vi "Draw Coord Point.vi"(5 "Marker Options":T3={"Color"=3784, "pen"={"Width"=2, "Style"=enum."Solid"}, "font"={"Font Name"="Arial", "Size"=16, "Strikeout?"=FALSE, "Italic?"=FALSE, "Underline?"=FALSE, "Outline?"=FALSE, "Shadow?"=FALSE, "Bold?"=FALSE, "FontColor"=3784}, "caption"=""}, 7 "radius":i16=5, 8 "error in (no error)":errorcluster, 10 "XY":T2, 11 "GarphView in":refnum<class "GarphView.lvclass">) -> (0 "error out":errorcluster, 3 "GarphView out":refnum<class "GarphView.lvclass">)   [LabVIEW 2020, in "GarphView.lvlib" / "GarphView.lvclass"]
uses:
  GarphView.lvclass
  Coords Point.ctl
  <vilib>/Utility/miscctls.llb/LVPoint32TypeDef.ctl
panel:
  out "Coords 2":T1
  out "Coords":T1
  out "XY Graph":cluster{"X":dbl, "Y":dbl}[](graph)
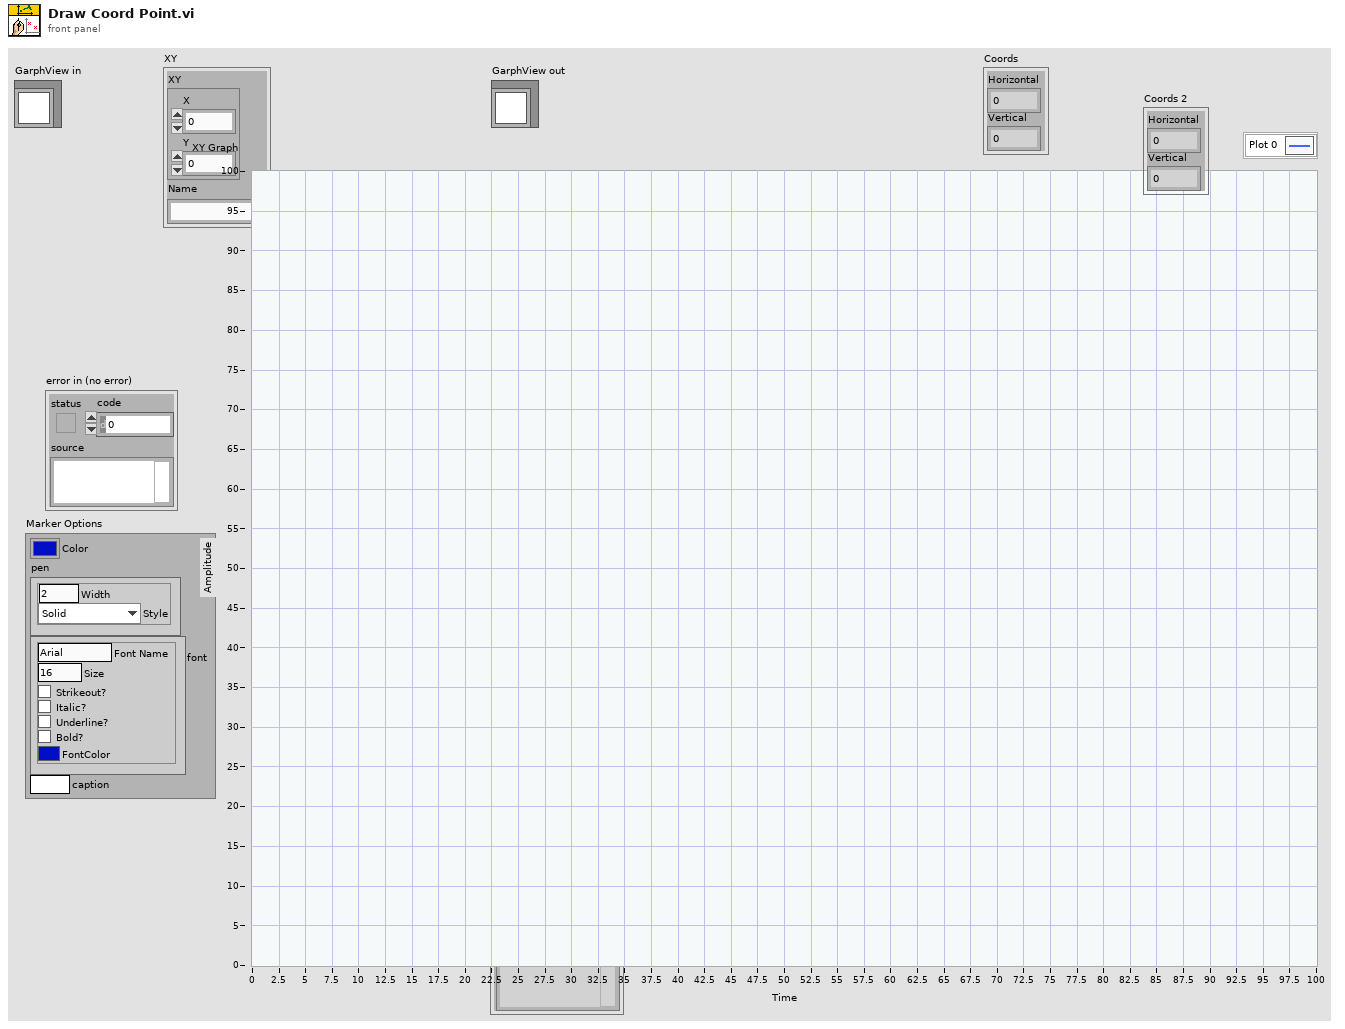
[diagram p1: front panel]
types:
  T1 = typedef "LVPoint32TypeDef.ctl" = cluster{"Horizontal":i32, "Vertical":i32}
  T2 = typedef "GarphView.lvlib/GarphView.lvclass/Coords Point.ctl" = cluster{"XY":cluster{"X":dbl, "Y":dbl}, "Name":string}
  T3 = cluster{"Color":u32, "pen":cluster{"Width":u16, "Style":enum32{"Solid", "Dash", "Dot", "DashDot", "DashDotDot"}}, "font":cluster{"Font Name":string, "Size":i16, "Strikeout?":bool, "Italic?":bool, "Underline?":bool, "Outline?":bool, "Shadow?":bool, "Bold?":bool, "FontColor":u32}, "caption":string}
  T4 = cluster{"Font Name:":string, "Size":i16, "Strikeout?":bool, "Italic?":bool, "Underline?":bool, "Outline?":bool, "Shadow?":bool, "Bold?":bool}
  T5 = enum16{"User-specified Font", "Application Font", "System Font", "Dialog Font"}
  T6 = typedef "LVRectTypeDef.ctl" = cluster{"Left":i16, "Top":i16, "Right":i16, "Bottom":i16}
  T7 = cluster{"Width":u16, "Style":enum32{"Solid", "Dash", "Dot", "DashDot", "DashDotDot"}}
  T8 = cluster{"Font Name":string, "Size":i16, "Strikeout?":bool, "Italic?":bool, "Underline?":bool, "Outline?":bool, "Shadow?":bool, "Bold?":bool, "FontColor":u32}
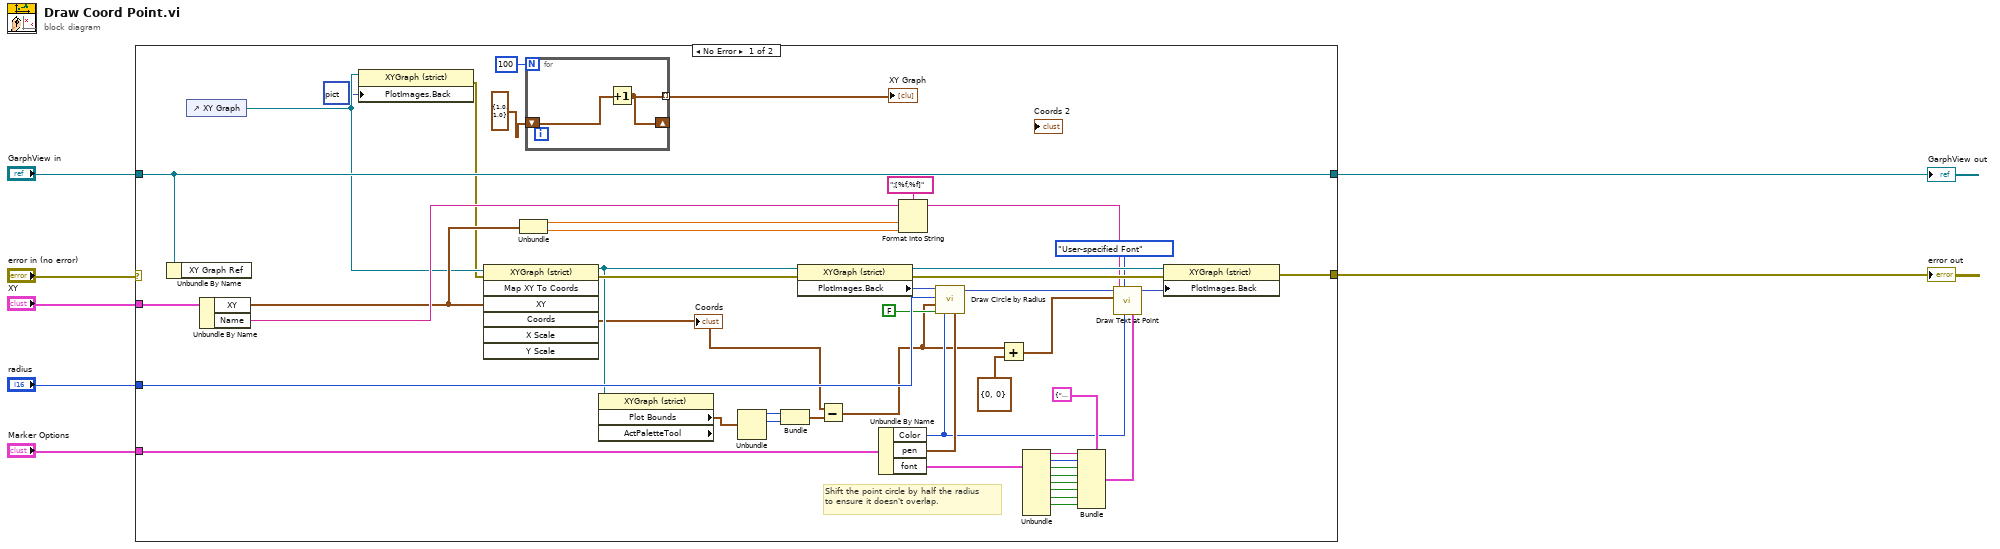
[diagram p0: block diagram]
diagram:
  n1 = case shown="No Error" "error in (no error)" {
    selector: "error in (no error)" -> [_ w58]
    tunnel: "Marker Options" -> [w54 _]
    tunnel: "GarphView in" -> [w49 w57]
    tunnel: "XY" -> [w25 _]
    tunnel: [w50 w58] -> w3
    tunnel: [w49 w57] -> w2
    tunnel: "radius" -> [w47 _]
    frame No Error {
      # "Shift the point circle by half the radius to ensure it doesn't overlap."
      n2 = Unbundle By Name(w49) -> ()  [unwired: 1 out]
      n3 = control-ref of="XY Graph"() -> (w20:refnum<vi>)
      n4 = Unbundle By Name(w25) -> ("XY"=w21:cluster{"X":dbl, "Y":dbl}, "Name"=w24:string)
      n5 = property class="XYGraph (strict)"(reference=w20, "PlotImages.Back"=picture data[5B] ("Plot Images:Back")) -> (error out=w18:errorcluster)  [unwired: 1 in, 1 out]
      n6 = invoke class="XYGraph (strict)" method="Map XY To Coords"(reference=w20, error in=w18, "XY"=w21) -> (reference out=w14:refnum<vi>, error out=w53:errorcluster, "Coords"=w9:T1)  [unwired: 4 in, 4 out]
      "Coords" <- w9
      n7 = Unbundle(w21) -> ("X"=w23:dbl, "Y"=w22:dbl)
      n8 = for {
        N: 100 -> [_]
        tunnel: [w56] -> w17 mode=indexing
        shift-right: [w56] -> _
        shift-left: cluster{"X":dbl, "Y":dbl} {"X"=1.0, "Y"=1.0} ("XY Graph") -> [w55]
        n9 = Increment(x=w55) -> (x+1=w56:cluster{"X":dbl, "Y":dbl})
      }
      "XY Graph" <- w17
      n10 = property on="Property Node" class="XYGraph (strict)" props=["Plot Bounds", "ActPaletteTool"](reference=w14) -> ("Plot Bounds"=w10:T6)  [unwired: 1 in, 3 out]
      n11 = Unbundle(w10) -> ("Left"=w12:i16, "Top"=w13:i16)  [unwired: 2 out]
      n12 = Bundle("Left"=w12, "Top"=w13) -> (w11:cluster{"Left":i16, "Top":i16})  [unwired: 1 in]
      n13 = property class="XYGraph (strict)"(reference=w14, error in=w53) -> (reference out=w52:refnum<vi>, error out=w51:errorcluster, "PlotImages.Back"=w48:picture)
      n14 = Subtract(x=w9, y=w11) -> (x-y=w8:T1)
      n15 = Unbundle By Name(w54) -> ("Color"=w26:u32, "pen"=w46:T7, "font"=w37:T8)
      n16 = Format Into String(format string=";[%f,%f]", initial string=w24, w23, w22) -> (resulting string=w27:string)  [unwired: 1 in, 1 out]
      n17 = call <vilib>:"Draw Circle by Radius.vi"("pen"=w46, "color(black)"=w26, "fill?(F)"=FALSE, "pixel center"=w8, "radius"=w47, "picture"=w48) -> ("new picture"=w39:picture)  [unwired: 5 in]
      n18 = Add(x=w8, y=T1 {"Horizontal"=0, "Vertical"=0} ("x+y")) -> (x+y=w44:T1)
      n19 = Unbundle(w37) -> ("Font Name"=w36:string, "Size"=w35:i16, "Strikeout?"=w34:bool, "Italic?"=w33:bool, "Underline?"=w32:bool, "Outline?"=w31:bool, "Shadow?"=w30:bool, "Bold?"=w29:bool)  [unwired: 1 out]
      n20 = Bundle(cluster=T4 {"Font Name:"="", "Size"=12, "Strikeout?"=FALSE, "Italic?"=FALSE, "Underline?"=FALSE, "Outline?"=FALSE, "Shadow?"=FALSE, "Bold?"=FALSE} ("[user-specified font]"), "Font Name:"=w36, "Size"=w35, "Strikeout?"=w34, "Italic?"=w33, "Underline?"=w32, "Outline?"=w31, "Shadow?"=w30, "Bold?"=w29) -> (w41:T4)
      n21 = call <vilib>:"Draw Text at Point.vi"("[user-specified font]"=w41, "text color(black)"=w26, "desired font(Application)"=T5."User-specified Font", "text"=w27, "origin"=w44, "picture"=w39) -> ("new picture"=w38:picture)  [unwired: 4 in, 1 out]
      n22 = property class="XYGraph (strict)"(reference=w52, error in=w51, "PlotImages.Back"=w38) -> (error out=w50:errorcluster)  [unwired: 1 out]
    }
    frame Error {
    }
  }
  "error out" <- w3
  "GarphView out" <- w2
